vi "String to I8.vi"(1 "String":string) -> (0 "I8":i8)   [LabVIEW 2011]
doc: "Convert string to number. Small VI to be block-diagram friendly.\n\nVersion 1.0 - 09/13/2013\n\nPhaeron, Inc.\nwww.phaeron.com\ninfo@phaeron.com"
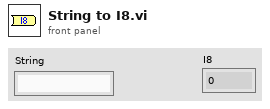
[diagram p1: front panel]
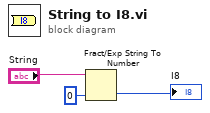
[diagram p0: block diagram]
diagram:
  n1 = Fract/Exp String To Number(string="String", default (0 dbl)=i8 0 ("default (0 DBL)")) -> (number=→"I8":i8)  [unwired: 2 in, 1 out]
